vi "SHOOTER.vi"(10 "argv":string[](array[string]), 11 "args":u8) -> ()   [LabVIEW 2012]
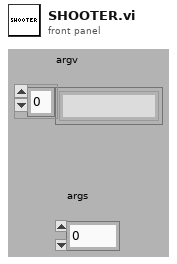
[diagram p1: front panel]
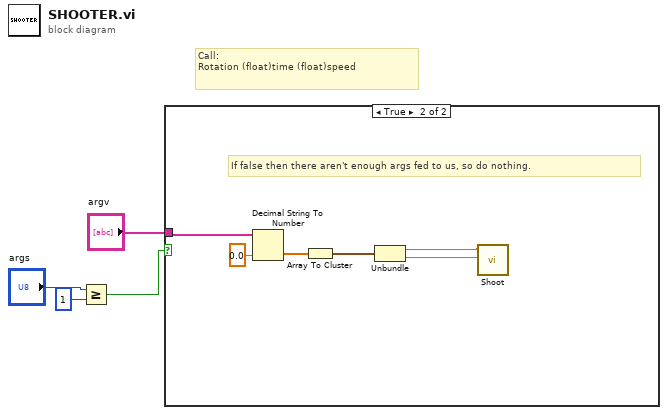
[diagram p0: block diagram]
diagram:
  # "Call:\nRotation (float)time (float)speed"
  n1 = Greater Or Equal?(x="args", y=u8 1) -> (x >= y?=w2:bool)
  n2 = case shown="True" w2 {
    tunnel: "argv" -> [_ w9]
    frame False {
    }
    frame True {
      # "If false then there aren't enough args fed to us, so do nothing."
      n3 = Decimal String To Number(string=w9, default (0L)=0.0 ("default (0 I32)")) -> (number=w7:dbl[])  [unwired: 2 out]
      n4 = Array To Cluster(array=w7) -> (cluster=w10:cluster{"[0]":dbl, "[1]":dbl})
      n5 = Unbundle(w10) -> ("[0]"=w6:dbl, "[1]"=w5:dbl)
      n6 = call "Shoot.vi"("User Input"=w5, "Numeric"=w6) -> ()  [unwired: 10 in]
    }
  }
